vi "TSM SSC DAQmx Timing.vi"(0 "DAQ TSM in":T1, 1 "Sample Mode":i32(ring)=10123 items=["Finite Samples"=10178, "Continuous Samples"=10123, "Hardware Timed Single Point"=12522], 2 "Samples":i32=1000, 5 "Sample Rate":dbl=1000.0 format="%0.2f", 7 "Source":tag, 9 "Active Edge":i32(ring)=10280 items=["Rising"=10280, "Falling"=10171], 11 "error in (no error)":errorcluster, 12 "Set Reference Clock Source?":bool, 13 "RefClk.Src":tag="PXIe_Clk100") -> (4 "DAQ TSM Out":T1, 15 "error out":errorcluster)   [LabVIEW 2020]
doc: "Sets the source of the Sample Clock, the rate of the Sample Clock, and the number of samples to acquire or generate.\nOptionally set the reference clock source."
uses:
  Pin Map/TSM DAQmx Multi-Task.ctl
  <vilib>/NI_TestStand_SemiconductorModule/NI_TestStand_Semiconductor_Module.lvlibp/PinMap/PinQueryContext/MultiplePinMultipleSessionQueryContext/MultiplePinMultipleSessionQueryContext.lvclass
  Pin Map/SSC DAQmx.ctl
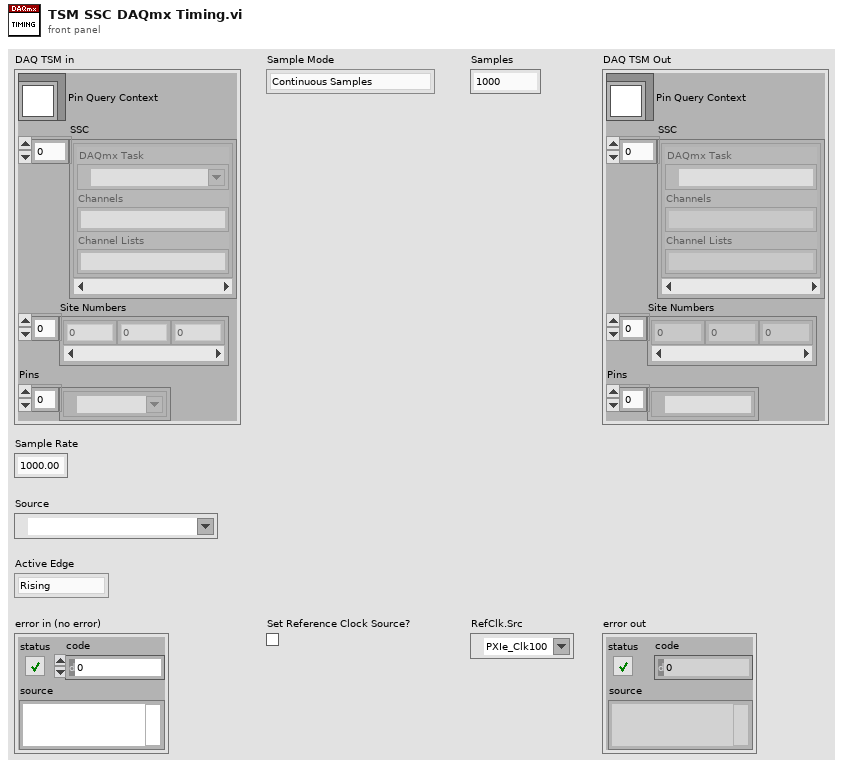
[diagram p1: front panel]
types:
  T1 = typedef "TSM DAQmx Multi-Task.ctl" = cluster{"Pin Query Context":refnum<class "MultiplePinMultipleSessionQueryContext.lvclass">, "SSC":T2[], "Site Numbers":i32[], "Pins":tag[]}
  T2 = typedef "SSC DAQmx.ctl" = cluster{"DAQmx Task ":refnum<k21>, "Channels":string, "Channel Lists":string}
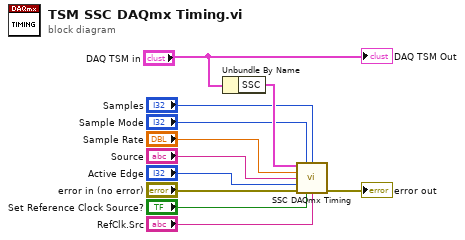
[diagram p0: block diagram]
diagram:
  n1 = Unbundle By Name("DAQ TSM in") -> ("SSC"=w9:T2[])
  n2 = call "SSC DAQmx Timing.vi"("DAQmx SSC in"=w9, "Sample Mode"="Sample Mode", "Samples"="Samples", "Sample Rate"="Sample Rate", "Source"="Source", "Active Edge"="Active Edge", "error in"="error in (no error)", "Set Reference Clock Source?"="Set Reference Clock Source?", "RefClk.Src"="RefClk.Src") -> ("error out"=→"error out":errorcluster)  [unwired: 5 in, 1 out]
  "DAQ TSM Out" <- "DAQ TSM in"
